vi "Write file name.vi"(8 "error in (no error)":errorcluster, 10 "suffix":string, 11 "Log File in":refnum<class "Events Log File.lvclass">) -> (0 "error out":errorcluster, 3 "Log File out":refnum<class "Events Log File.lvclass">)   [LabVIEW 2018, in "Events Log File.lvclass"]
uses:
  Events Log File.lvclass
  Events Log File.lvclass/Events Log File.ctl
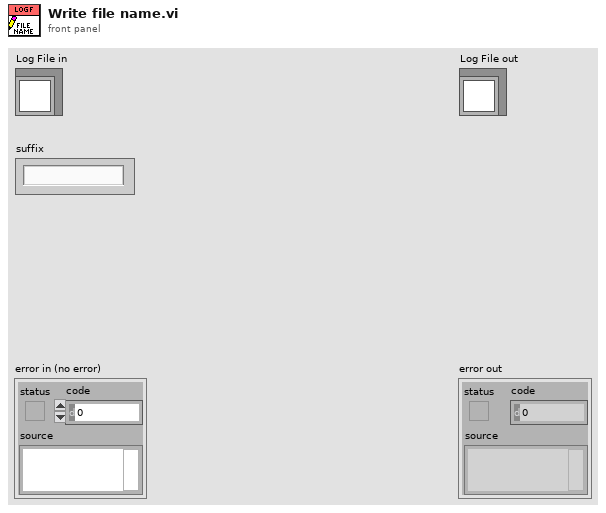
[diagram p1: front panel]
types:
  T1 = typedef "LVDateTimeRec.ctl" = cluster{"fractional second":dbl, "second":i32, "minute":i32, "hour":i32, "day of month":i32, "month":i32, "year":i32, "day of week":i32, "day of year":i32, "DST":i32}
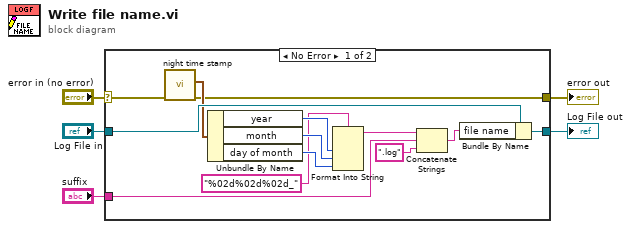
[diagram p0: block diagram]
diagram:
  n1 = case shown="No Error" "error in (no error)" {
    selector: "error in (no error)" -> [w11 w19]
    tunnel: [w6 w19] -> w4
    tunnel: [w17 w20] -> w2
    tunnel: "Log File in" -> [w18 w20]
    tunnel: "suffix" -> [w9 _]
    frame No Error {
      n2 = call "night time stamp.vi"("error in (no error)"=w11) -> ("error out"=w6:errorcluster, "date time rec"=w12:T1)  [unwired: 9 in]
      n3 = Unbundle By Name(w12) -> ("year"=w16:i32, "month"=w15:i32, "day of month"=w14:i32)
      n4 = Format Into String(format string="%02d%02d%02d_", w16, w15, w14) -> (resulting string=w10:string)  [unwired: 2 in, 1 out]
      n5 = Concatenate Strings(w10, w9, ".log" ("string")) -> (w7:string)
      n6 = Bundle By Name(cluster=w18, "file name"=w7) -> (w17:refnum<class "Events Log File.lvclass">)
    }
    frame Error {
    }
  }
  "error out" <- w4
  "Log File out" <- w2
